vi "get_around_obstacle.vi"(9 "Boat location":T1 {"North" format="%#_10f"; "East" format="%#_8f"}, 10 "Obstacle array":refnum<class "Obstacle.lvclass">[](array[class]), 11 "Waypoint queue":refnum<queue>) -> (2 "Added intermediate point?":bool, 3 "Waypoint queue out":refnum<queue>)   [LabVIEW 2013]
uses:
  Classes/Waypoint/Waypoint.lvclass
  Classes/Obstacle/Obstacle.lvclass
  Data/TypeDefs/UTM Location.ctl
  Utilities/Math/Angles/Angle/Angle.lvclass
panel:
  in  "Step size for angle sweep":dbl=5.0
  out "Heading from boat to waypoint #1":dbl
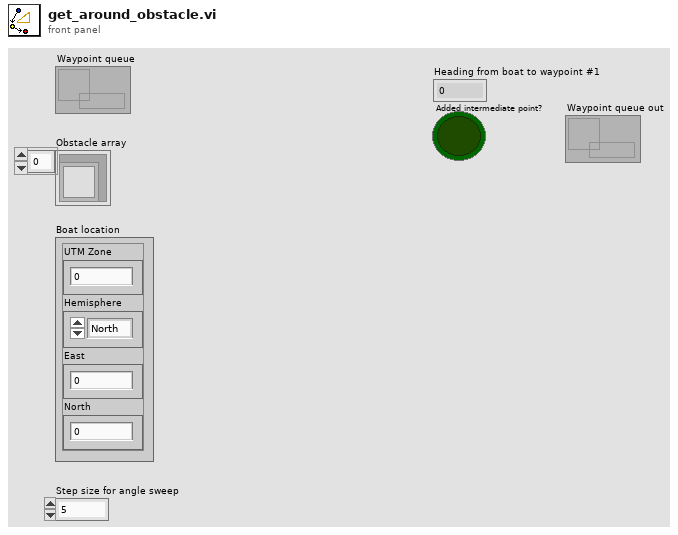
[diagram p1: front panel]
types:
  T1 = typedef "UTM Location.ctl" = cluster{"UTM Zone":dbl, "Hemisphere":enum16{"North", "South"}, "East":dbl, "North":dbl}
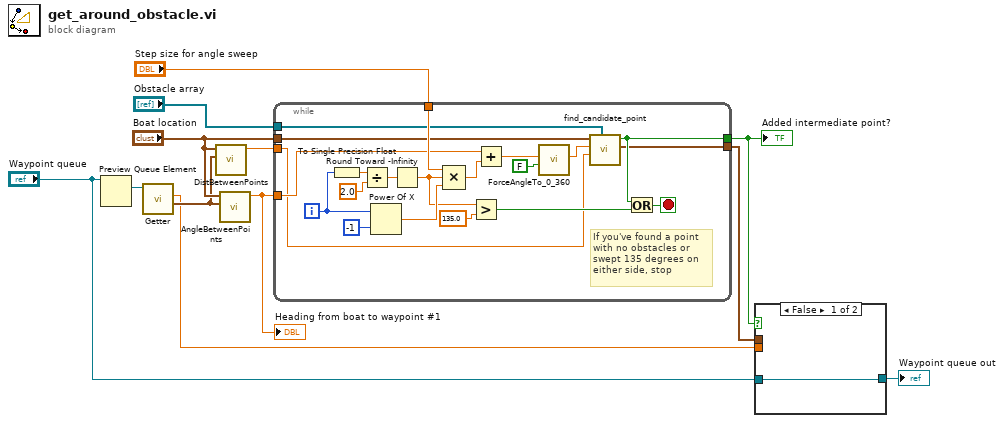
[diagram p0: block diagram]
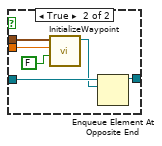
[diagram p2: hidden frame]
diagram:
  n1 = Preview Queue Element(queue="Waypoint queue") -> (element=w12:refnum<class "Waypoint.lvclass">)  [unwired: 2 in, 3 out]
  n2 = call "Getter.vi"("Waypoint In"=w12) -> ("Coords"=w7:T1, "Tolerance (meters?)"=w3:dbl)  [unwired: 6 in, 3 out]
  n3 = call "DistBetweenPoints.vi"("UTM Location 2"=w7, "UTM Location 1"="Boat location") -> ("Distance from 1 to 2"=w6:dbl)  [unwired: 9 in]
  n4 = call "AngleBetweenPoints.vi"("Point 2"=w7, "Point 1"="Boat location") -> ("Angle from P1 to P2"=w11:dbl)  [unwired: 9 in]
  "Heading from boat to waypoint #1" <- w11
  n5 = while {
    tunnel: w11 -> [w23]
    tunnel: "Step size for angle sweep" -> [w28]
    tunnel: "Boat location" -> [w19]
    tunnel: "Obstacle array" -> [w18]
    tunnel: w6 -> [w15]
    tunnel: [w14] -> w5
    tunnel: [w13] -> w4
    i -> [w32]
    stop <- w24 stop-if-true
    # "If you've found a point with no obstacles or swept 135 degrees on either side, stop"
    n6 = To Single Precision Float(number=w32) -> (single precision float=w31:sgl)
    n7 = Divide(x=w31, y=sgl 2.0) -> (x/y=w29:sgl)
    n8 = Power Of X(1:-1 ("x"), 2:w32) -> (0:w27:dbl)
    n9 = Round Toward -Infinity(1:w29) -> (0:w26:sgl)
    n10 = Compound Arithmetic op=MULTIPLY(w28, w26, w27) -> (w22:dbl)
    n11 = Greater?(x=w26, y=sgl 135.0) -> (0:w17:bool)
    n12 = Add(x=w23, y=w22) -> (x+y=w20:dbl)
    n13 = call "ForceAngleTo_0_360.vi"("Use angle class? (T)"=FALSE, "Angle in"=w20) -> ("Forced Angle"=w16:dbl)  [unwired: 7 in, 2 out]
    n14 = call "find_candidate_point.vi"("Obstacle array"=w18, "Distance from boat to waypoint"=w15, "Candidate heading"=w16, "Boat location"=w19) -> ("Intermediate Point"=w13:T1, "Point good?"=w14:bool)  [unwired: 6 in]
    n15 = Or(x=w14, y=w17) -> (x .or. y?=w24:bool)
  }
  "Added intermediate point?" <- w5
  n16 = case shown="False" w5 {
    tunnel: w4 -> [_ w38]
    tunnel: w3 -> [_ w39]
    tunnel: "Waypoint queue" -> [w34 w37]
    tunnel: [w34 w35] -> w1
    frame False {
    }
    frame True {
      n17 = call "InitializeWaypoint.vi"("Done? (F)"=FALSE, "Tolerance (meters?) (0)"=w39, "Coords"=w38) -> ("Waypoint Out"=w36:refnum<class "Waypoint.lvclass">)  [unwired: 8 in]
      n18 = Enqueue Element At Opposite End(queue=w37, element=w36) -> (queue out=w35:refnum<queue>)  [unwired: 2 in, 2 out]
    }
  }
  "Waypoint queue out" <- w1
